vi "Test jsObject Array.vi"(8 "error in (no error)":errorcluster, 9 "TESTS (none)":T1[](array[typedef]), 10 "Tests jsObject Array Name (\"TESTS\")":string="TESTS", 11 "Previous String (\"\")":string) -> (0 "error out":errorcluster, 2 "Tests jsObject Array":string, 3 "Test Definition":string)   [LabVIEW 2011]
uses:
  Test Record.ctl
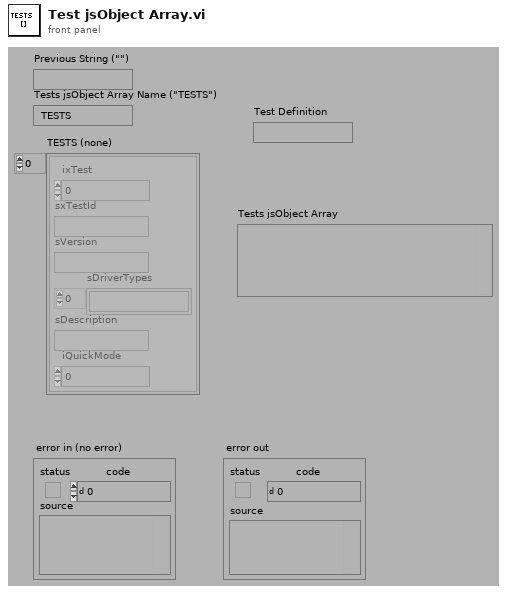
[diagram p1: front panel]
types:
  T1 = typedef "Test Record.ctl" = cluster{"ixTest":i32, "sxTestId":string, "sVersion":string, "sDriverTypes":string[], "sDescription":string, "iQuickMode":i32}
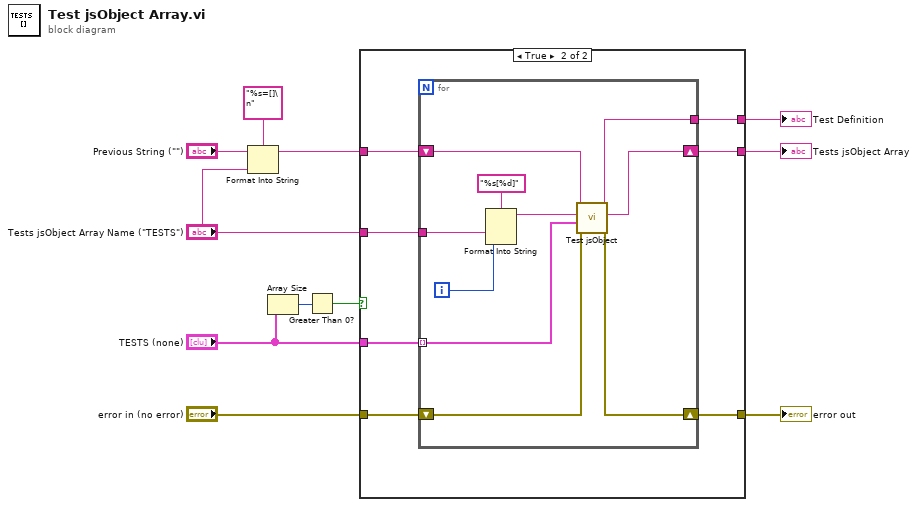
[diagram p0: block diagram]
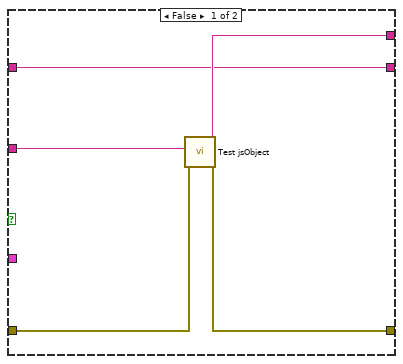
[diagram p2: hidden frame]
diagram:
  n1 = Format Into String(format string="%s=[]\n", initial string="Previous String (\"\")", "Tests jsObject Array Name (\"TESTS\")") -> (resulting string=w10:string)  [unwired: 1 in, 1 out]
  n2 = Array Size(array="TESTS (none)") -> (size(s)=w9:i32)
  n3 = Greater Than 0?(x=w9) -> (x > 0?=w8:bool)
  n4 = case shown="True" w8 {
    tunnel: w10 -> [w12 w23]
    tunnel: "error in (no error)" -> [w16 w22]
    tunnel: [w12 w21] -> w4
    tunnel: [w15 w20] -> w3
    tunnel: "Tests jsObject Array Name (\"TESTS\")" -> [w13 w19]
    tunnel: [w14 w18] -> w5
    tunnel: "TESTS (none)" -> [_ w17]
    frame False {
      n5 = call "Test jsObject.vi"("error in (no error)"=w16, "Step jsObject Name (\"\")"=w13) -> ("error out"=w15:errorcluster, "TEST definition"=w14:string)  [unwired: 2 in, 6 out]
    }
    frame True {
      n6 = for {
        tunnel: w17 -> [w26] mode=indexing
        shift-right: [w24] -> w21
        shift-left: w23 -> [w33]
        shift-right: [w31] -> w20
        shift-left: w22 -> [w32]
        tunnel: w19 -> [w28]
        tunnel: [w25] -> w18
        i -> [w27]
        n7 = Format Into String(format string="%s[%d]", w28, w27) -> (resulting string=w29:string)  [unwired: 2 in, 1 out]
        n8 = call "Test jsObject.vi"("error in (no error)"=w32, "Test Record (empty)"=w26, "Step jsObject Name (\"\")"=w29, "Previous String (\"\")"=w33) -> ("error out"=w31:errorcluster, "TEST jsObject"=w24:string, "TEST definition"=w25:string)  [unwired: 5 out]
      }
    }
  }
  "Tests jsObject Array" <- w4
  "error out" <- w3
  "Test Definition" <- w5
